vi "testCreateMultipleTcpIpConnectionsServersAandB.vi"(8 "error in":errorcluster) -> (0 "error out":errorcluster)   [LabVIEW 2018]
uses:
  src/FactoryTcpServer/FactoryTcpServer.lvclass
  <vilib>/addons/_JKI Toolkits/Caraya/classes/Assert/Assert Equal Value_Variant.vi
  src/TcpServer/TcpServer.lvclass
  <vilib>/addons/_JKI Toolkits/Caraya/classes/Test/Test.lvclass
  <vilib>/addons/_JKI Toolkits/Caraya/classes/Assert/Assert.lvclass
panel:
  out "Run Server B error":errorcluster
  out "Run Server A error":errorcluster
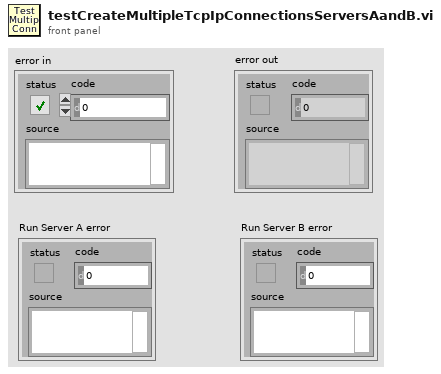
[diagram p1: front panel]
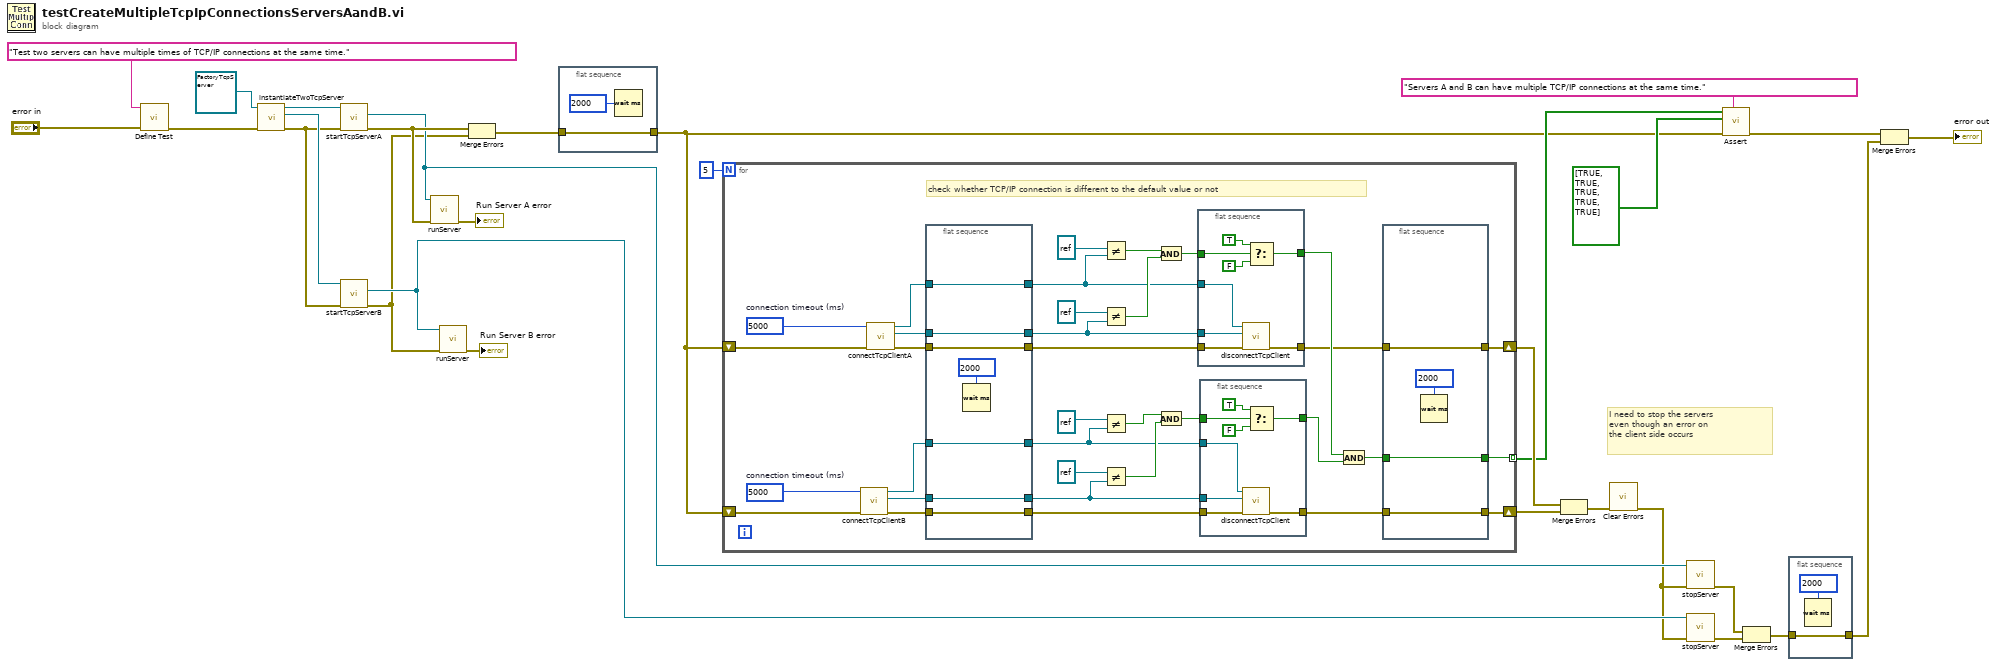
[diagram p0: block diagram]
diagram:
  # "I need to stop the servers \neven though an error on \nthe client side occurs"
  n1 = call <vilib>:"Define Test.vi"("error in (no error)"="error in", "Label (VI Title)"="Test two servers can have multiple times of TCP/IP connections at the same time.") -> ("error out"=w5:errorcluster)  [unwired: 9 in]
  n2 = call "instantiateTwoTcpServer.vi"("error in (no error)"=w5, "FactoryTcpServer in"=refnum<class "FactoryTcpServer.lvclass"> refnum) -> ("error out"=w1:errorcluster, "TcpServer 2 out"=w2:refnum<class "TcpServer.lvclass">, "TcpServer 1 out"=w3:refnum<class "TcpServer.lvclass">)  [unwired: 6 in, 1 out]
  n3 = call "startTcpServerA.vi"("error in (no error)"=w1, "TcpServer.lvclass"=w3) -> ("error out"=w27:errorcluster, "TcpServer out"=w26:refnum<class "TcpServer.lvclass">)  [unwired: 7 in, 1 out]
  n4 = call "startTcpServerB.vi"("error in (no error)"=w1, "TcpServer.lvclass"=w2) -> ("error out"=w8:errorcluster, "TcpServer out"=w22:refnum<class "TcpServer.lvclass">)  [unwired: 7 in, 1 out]
  n5 = call "runServer.vi"("error in (no error)"=w27, "TcpServer in"=w26) -> ("error out (no error)"=→"Run Server A error":errorcluster)  [unwired: 8 in, 1 out]
  n6 = call "runServer.vi"("error in (no error)"=w8, "TcpServer in"=w22) -> ("error out (no error)"=→"Run Server B error":errorcluster)  [unwired: 8 in, 1 out]
  n7 = Merge Errors(w27, w8) -> (w9:errorcluster)
  n8 = flat-sequence {
    tunnel: w9 -> [w30]
    tunnel: [w30] -> w12
    frame #0 {
      n9 = Wait (ms)(milliseconds to wait=u32 2000) -> ()  [unwired: 1 out]
    }
  }
  n10 = for {
    N: 5 -> [_]
    tunnel: [w39] -> w15 mode=indexing
    shift-right: [w37] -> w21
    shift-left: w12 -> [w44]
    shift-right: [w36] -> w20
    shift-left: w12 -> [w43]
    w32 = 5000  # connection timeout (ms)
    w33 = 5000  # connection timeout (ms)
    # "check whether TCP/IP connection is different to the default value or not"
    n11 = call "connectTcpClientB.vi"("error in (no error)"=w43, "connection timeout (ms)"=w32) -> ("error out"=w45:errorcluster, "tel connection ID B out"=w46:refnum<k5>, "cmd connection ID B out"=w47:refnum<k5>)  [unwired: 7 in]
    n12 = call "connectTcpClientA.vi"("error in (no error)"=w44, "connection timeout (ms)"=w33) -> ("error out"=w48:errorcluster, "tel connection ID A out"=w49:refnum<k5>, "cmd connection ID A out"=w50:refnum<k5>)  [unwired: 7 in]
    n13 = flat-sequence {
      tunnel: [w92] -> w56
      tunnel: w50 -> [w92]
      tunnel: [w91] -> w55
      tunnel: w49 -> [w91]
      tunnel: [w90] -> w54
      tunnel: w48 -> [w90]
      tunnel: [w89] -> w53
      tunnel: w47 -> [w89]
      tunnel: [w88] -> w52
      tunnel: w46 -> [w88]
      tunnel: w45 -> [w86]
      tunnel: [w86] -> w42
      frame #0 {
        n14 = Wait (ms)(milliseconds to wait=u32 2000) -> ()  [unwired: 1 out]
      }
    }
    n15 = Not Equal?(x=refnum<k5> refnum ("connection ID"), y=w56) -> (x != y?=w61:bool)
    n16 = Not Equal?(x=refnum<k5> refnum ("connection ID"), y=w55) -> (x != y?=w60:bool)
    n17 = Not Equal?(x=refnum<k5> refnum ("connection ID"), y=w53) -> (x != y?=w59:bool)
    n18 = Not Equal?(x=refnum<k5> refnum ("connection ID"), y=w52) -> (x != y?=w58:bool)
    n19 = Compound Arithmetic op=AND(w61, w60) -> (w57:bool)
    n20 = Compound Arithmetic op=AND(w59, w58) -> (w35:bool)
    n21 = flat-sequence {
      tunnel: w57 -> [w81]
      tunnel: w56 -> [w80]
      tunnel: w55 -> [w79]
      tunnel: w54 -> [w78]
      tunnel: [w77] -> w51
      tunnel: [w76] -> w41
      frame #0 {
        n22 = call "disconnectTcpClient.vi"("error in (no error)"=w78, "tel connection ID in"=w79, "cmd connection ID in"=w80) -> ("error out"=w76:errorcluster)  [unwired: 8 in]
        n23 = Select(t=TRUE, s=w81, f=FALSE) -> (s? t:f=w77:bool)
      }
    }
    n24 = flat-sequence {
      tunnel: w53 -> [w73]
      tunnel: w52 -> [w72]
      tunnel: w42 -> [w71]
      tunnel: [w70] -> w40
      tunnel: w35 -> [w67]
      tunnel: [w66] -> w34
      frame #0 {
        n25 = call "disconnectTcpClient.vi"("error in (no error)"=w71, "tel connection ID in"=w72, "cmd connection ID in"=w73) -> ("error out"=w70:errorcluster)  [unwired: 8 in]
        n26 = Select(t=TRUE, s=w67, f=FALSE) -> (s? t:f=w66:bool)
      }
    }
    n27 = Compound Arithmetic op=AND(w51, w34) -> (w38:bool)
    n28 = flat-sequence {
      tunnel: [w85] -> w37
      tunnel: w41 -> [w85]
      tunnel: w40 -> [w83]
      tunnel: [w83] -> w36
      tunnel: [w82] -> w39
      tunnel: w38 -> [w82]
      frame #0 {
        n29 = Wait (ms)(milliseconds to wait=u32 2000) -> ()  [unwired: 1 out]
      }
    }
  }
  n30 = Merge Errors(w21, w20) -> (w7:errorcluster)
  n31 = call <vilib>:"Clear Errors.vi"("error in (no error)"=w7) -> ("error out"=w6:errorcluster)  [unwired: 5 in, 1 out]
  n32 = call "stopServer.vi"("error in (no error)"=w6, "tcpServer in"=w26) -> ("error out"=w19:errorcluster)  [unwired: 8 in, 1 out]
  n33 = call "stopServer.vi"("error in (no error)"=w6, "tcpServer in"=w22) -> ("error out"=w18:errorcluster)  [unwired: 8 in, 1 out]
  n34 = call-poly <vilib>:"Assert.vi"("Label"="Servers A and B can have multiple TCP/IP connections at the same time.", "error in (no error)"=w12, "Y"=bool[] [TRUE, TRUE, TRUE, TRUE, TRUE], "X"=w15) -> ("error out"=w11:errorcluster)  [unwired: 7 in]
  n35 = Merge Errors(w19, w18) -> (w17:errorcluster)
  n36 = flat-sequence {
    tunnel: w17 -> [w93]
    tunnel: [w93] -> w10
    frame #0 {
      n37 = Wait (ms)(milliseconds to wait=u32 2000) -> ()  [unwired: 1 out]
    }
  }
  n38 = Merge Errors(w11, w10) -> (→"error out":errorcluster)
